vi "rfrobot.vi"() -> ()   [LabVIEW 2014]
uses:
  <vilib>/LabVIEW Hacker/LINX/Public/Peripherals/Digital/Digital Write 1 Chan.vi
  <vilib>/LabVIEW Hacker/LINX/Private/Type Defs/User Platform.ctl
  <vilib>/LabVIEW Hacker/LINX/Private/Type Defs/Interface.ctl
panel:
  in  "Boolean 4":bool
  in  "Boolean 3":bool
  in  "Boolean 2":bool
  in  "Boolean":bool
  in  "stop":bool
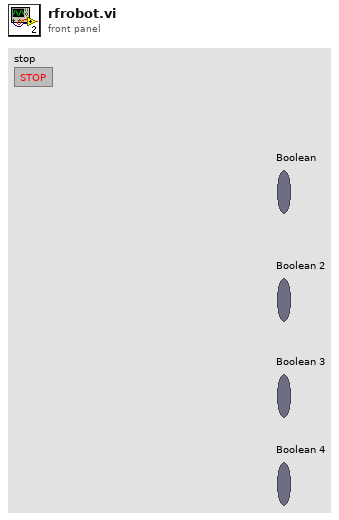
[diagram p1: front panel]
types:
  T1 = typedef "LVH-LINX.lvlib/Interface.ctl" = enum16{"Serial", "TCP"}
  T2 = typedef "LVH-LINX.lvlib/User Platform.ctl" = enum16{"Default", "LINX", "myRIO"}
  T3 = typedef "LVH-LINX.lvlib/LINX Ref.ctl" = cluster{"Platform":T4, "Interface":T1, "LINX Device Config":T5}
  T4 = typedef "LVH-LINX.lvlib/Platform.ctl" = enum16{"LINX", "myRIO"}
  T5 = typedef "LVH-LINX.lvlib/Device.lvlib/LINX Device Config.ctl" = cluster{"Interface":T1, "COM Port":refnum<visa-resource-name>, "TCP Configuration":T6, "Device Family":T7, "Device ID":u8, "Device Name":string, "TCP Ref":refnum<k5>}
  T6 = typedef "LVH-LINX.lvlib/Device.lvlib/TCP Config.ctl" = cluster{"IP Address":string, "Port":u16}
  T7 = typedef "LVH-LINX.lvlib/Device Family.ctl" = enum8{"National Instruments", "Digilent", "Arduino"}
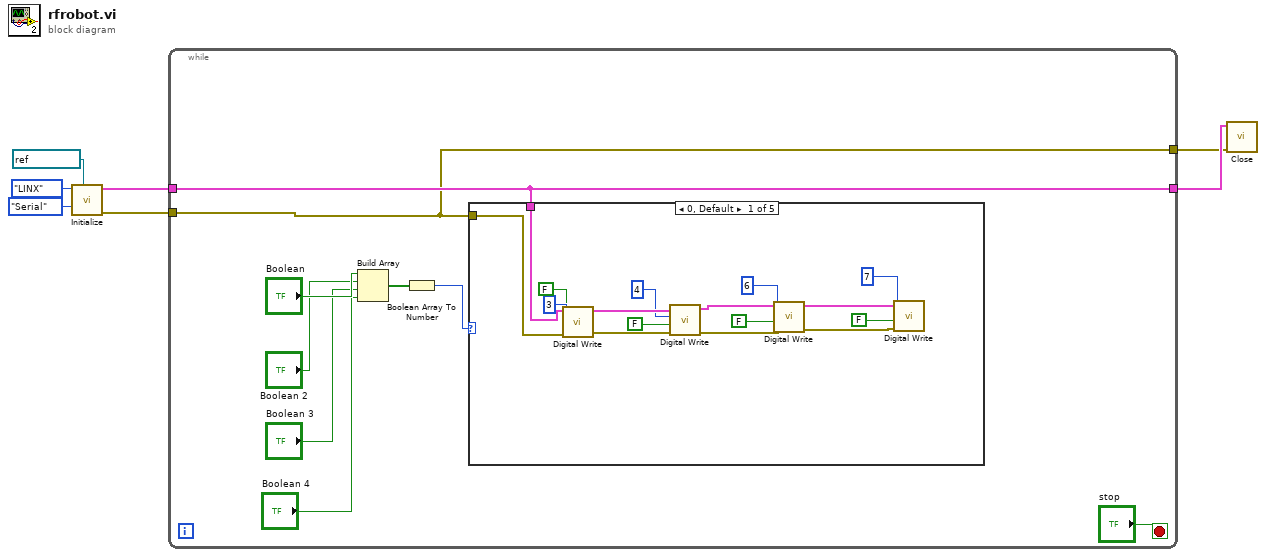
[diagram p0: block diagram]
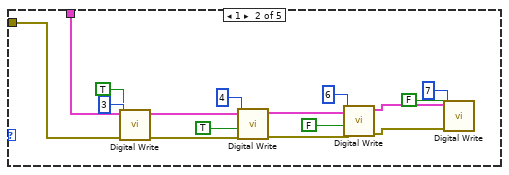
[diagram p2: hidden frame]
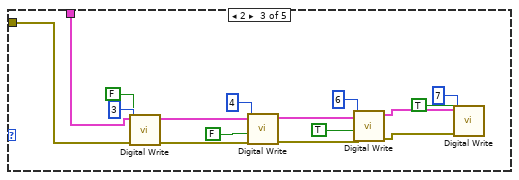
[diagram p3: hidden frame]
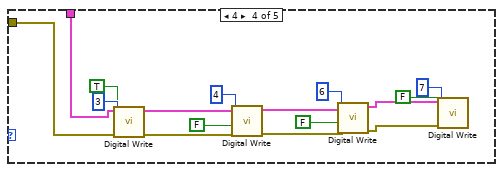
[diagram p4: hidden frame]
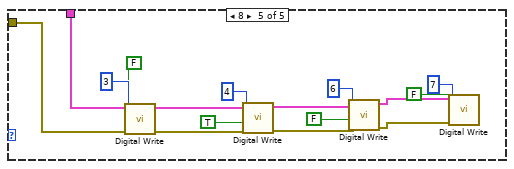
[diagram p5: hidden frame]
diagram:
  n1 = call <vilib>:"Initialize.vi"("Serial Port"=refnum<visa-resource-name> "COM17", "Interface"=Interface."Serial", "Platform"=User_Platform."LINX") -> ("Error Out"=w6:errorcluster, "LINX Ref"=w7:T3)  [unwired: 6 in, 1 out]
  n2 = while {
    tunnel: w7 -> [w10]
    tunnel: w6 -> [w9]
    tunnel: [w10] -> w5
    tunnel: [w9] -> w4
    stop <- "stop" stop-if-true
    n3 = Build Array("Boolean", "Boolean 2", "Boolean 3", "Boolean 4") -> (w11:bool[])
    n4 = Boolean Array To Number(Boolean array=w11) -> (number=w8:u32)
    n5 = case shown="0, Default" w8 {
      tunnel: w10 -> [w18 w42 w50 w66 w82]
      tunnel: w9 -> [w17 w41 w49 w65 w81]
      frame 0, Default {
        n6 = call-poly <vilib>:"Digital Write.vi"("Error In"=w17, "Output Value"=FALSE, "DO Channel"=u8 3, "LINX Resource"=w18) -> ("Error Out"=w31:errorcluster, "LINX Resource"=w32:T3)  [unwired: 6 in]
        n7 = call-poly <vilib>:"Digital Write.vi"("Error In"=w31, "Output Value"=FALSE, "DO Channel"=u8 4, "LINX Resource"=w32) -> ("Error Out"=w29:errorcluster, "LINX Resource"=w30:T3)  [unwired: 6 in]
        n8 = call-poly <vilib>:"Digital Write.vi"("Error In"=w29, "Output Value"=FALSE, "DO Channel"=u8 6, "LINX Resource"=w30) -> ("Error Out"=w27:errorcluster, "LINX Resource"=w28:T3)  [unwired: 6 in]
        n9 = call-poly <vilib>:"Digital Write.vi"("Error In"=w27, "Output Value"=FALSE, "DO Channel"=u8 7, "LINX Resource"=w28) -> ()  [unwired: 6 in, 2 out]
      }
      frame 1 {
        n10 = call-poly <vilib>:"Digital Write.vi"("Error In"=w41, "Output Value"=TRUE, "DO Channel"=u8 3, "LINX Resource"=w42) -> ("Error Out"=w45:errorcluster, "LINX Resource"=w48:T3)  [unwired: 6 in]
        n11 = call-poly <vilib>:"Digital Write.vi"("Error In"=w45, "Output Value"=TRUE, "DO Channel"=u8 4, "LINX Resource"=w48) -> ("Error Out"=w44:errorcluster, "LINX Resource"=w47:T3)  [unwired: 6 in]
        n12 = call-poly <vilib>:"Digital Write.vi"("Error In"=w44, "Output Value"=FALSE, "DO Channel"=u8 6, "LINX Resource"=w47) -> ("Error Out"=w43:errorcluster, "LINX Resource"=w46:T3)  [unwired: 6 in]
        n13 = call-poly <vilib>:"Digital Write.vi"("Error In"=w43, "Output Value"=FALSE, "DO Channel"=u8 7, "LINX Resource"=w46) -> ()  [unwired: 6 in, 2 out]
      }
      frame 2 {
        n14 = call-poly <vilib>:"Digital Write.vi"("Error In"=w49, "Output Value"=FALSE, "DO Channel"=u8 3, "LINX Resource"=w50) -> ("Error Out"=w61:errorcluster, "LINX Resource"=w64:T3)  [unwired: 6 in]
        n15 = call-poly <vilib>:"Digital Write.vi"("Error In"=w61, "Output Value"=FALSE, "DO Channel"=u8 4, "LINX Resource"=w64) -> ("Error Out"=w60:errorcluster, "LINX Resource"=w63:T3)  [unwired: 6 in]
        n16 = call-poly <vilib>:"Digital Write.vi"("Error In"=w60, "Output Value"=TRUE, "DO Channel"=u8 6, "LINX Resource"=w63) -> ("Error Out"=w59:errorcluster, "LINX Resource"=w62:T3)  [unwired: 6 in]
        n17 = call-poly <vilib>:"Digital Write.vi"("Error In"=w59, "Output Value"=TRUE, "DO Channel"=u8 7, "LINX Resource"=w62) -> ()  [unwired: 6 in, 2 out]
      }
      frame 4 {
        n18 = call-poly <vilib>:"Digital Write.vi"("Error In"=w65, "Output Value"=TRUE, "DO Channel"=u8 3, "LINX Resource"=w66) -> ("Error Out"=w77:errorcluster, "LINX Resource"=w80:T3)  [unwired: 6 in]
        n19 = call-poly <vilib>:"Digital Write.vi"("Error In"=w77, "Output Value"=FALSE, "DO Channel"=u8 4, "LINX Resource"=w80) -> ("Error Out"=w76:errorcluster, "LINX Resource"=w79:T3)  [unwired: 6 in]
        n20 = call-poly <vilib>:"Digital Write.vi"("Error In"=w76, "Output Value"=FALSE, "DO Channel"=u8 6, "LINX Resource"=w79) -> ("Error Out"=w75:errorcluster, "LINX Resource"=w78:T3)  [unwired: 6 in]
        n21 = call-poly <vilib>:"Digital Write.vi"("Error In"=w75, "Output Value"=FALSE, "DO Channel"=u8 7, "LINX Resource"=w78) -> ()  [unwired: 6 in, 2 out]
      }
      frame 8 {
        n22 = call-poly <vilib>:"Digital Write.vi"("Error In"=w81, "Output Value"=FALSE, "DO Channel"=u8 3, "LINX Resource"=w82) -> ("Error Out"=w93:errorcluster, "LINX Resource"=w96:T3)  [unwired: 6 in]
        n23 = call-poly <vilib>:"Digital Write.vi"("Error In"=w93, "Output Value"=TRUE, "DO Channel"=u8 4, "LINX Resource"=w96) -> ("Error Out"=w92:errorcluster, "LINX Resource"=w95:T3)  [unwired: 6 in]
        n24 = call-poly <vilib>:"Digital Write.vi"("Error In"=w92, "Output Value"=FALSE, "DO Channel"=u8 6, "LINX Resource"=w95) -> ("Error Out"=w91:errorcluster, "LINX Resource"=w94:T3)  [unwired: 6 in]
        n25 = call-poly <vilib>:"Digital Write.vi"("Error In"=w91, "Output Value"=FALSE, "DO Channel"=u8 7, "LINX Resource"=w94) -> ()  [unwired: 6 in, 2 out]
      }
    }
  }
  n26 = call <vilib>:"Close.vi"("Error In"=w4, "LINX Resource"=w5) -> ()  [unwired: 8 in, 2 out]
